vi "Load-Save Color Palette List.vi"(6 "Load (F)/Save":bool, 8 "error in (no error)":errorcluster, 9 "[Color Palette Name] in":string[](array[string]), 10 "Color Palette Target":string="Color Lists", 11 "ini File Refnum in":T1) -> (0 "error out":errorcluster, 1 "[Color Palette Name] out":string[](array[string]), 3 "ini File Refnum out":T1)   [LabVIEW 2021, in "Palette.lvlib"]
uses:
  <vilib>/Utility/config.llb/Config Data RefNum.ctl
  Palette.lvlib
  Variant/Variant to Data/Variant to [String].vi
  <userlib>/_OpenG.lib/variantconfig/variantconfig.llb/openg_variant_configuration_file.lvlib
  Variant/Variant to Data/Variant to Data.lvlib
  <vilib>/Utility/config.llb/NI_LVConfig.lvlib
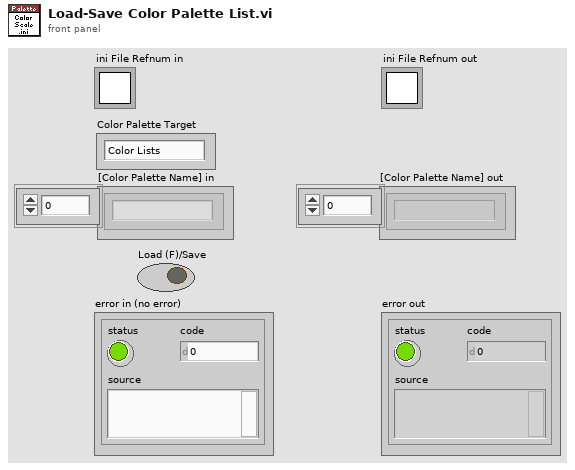
[diagram p1: front panel]
types:
  T1 = typedef "NI_LVConfig.lvlib/Config Data RefNum.ctl" = refnum<k1>
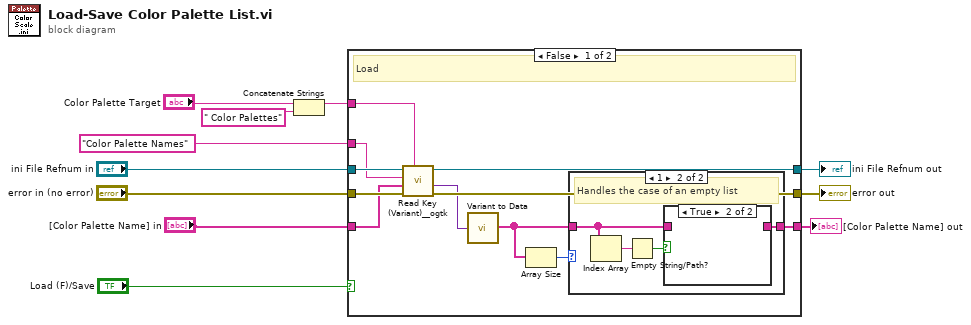
[diagram p0: block diagram]
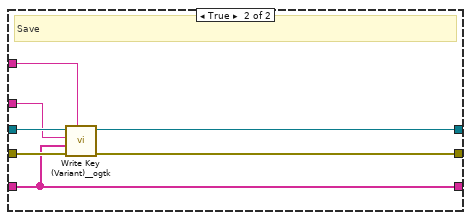
[diagram p4: hidden frame]
diagram:
  n1 = Concatenate Strings("Color Palette Target", " Color Palettes" ("string")) -> (w2:string)
  n2 = case shown="False" "Load (F)/Save" {
    tunnel: "ini File Refnum in" -> [w22 w35]
    tunnel: [w19 w34] -> w8
    tunnel: [w18 w33] -> w6
    tunnel: "error in (no error)" -> [w21 w30]
    tunnel: w2 -> [w17 w32]
    tunnel: "Color Palette Names" ("key (optional)") -> [w20 w31]
    tunnel: "[Color Palette Name] in" -> [w16 w29]
    tunnel: [w12 w29] -> w3
    frame False {
      # "Load"
      n3 = call <userlib>:"Read Key (Variant)__ogtk.vi"("section"=w17, "error in (no error)"=w21, "type"=w16, "key (optional)"=w20, "refnum"=w22) -> ("error out"=w18:errorcluster, "key-value"=w15:variant, "refnum out"=w19:T1)  [unwired: 3 in, 1 out]
      n4 = call-poly "Variant to Data.vi"("Variant"=w15) -> ("String Array"=w13:string[])  [unwired: 8 in]
      n5 = Array Size(array=w13) -> (size(s)=w14:i32)
      n6 = case shown="1" w14 {
        tunnel: w13 -> [w23 w25]
        tunnel: [w23 w24] -> w12
        frame 0, Default {
        }
        frame 1 {
          # "Handles the case of an empty list"
          n7 = Index Array(array=w25) -> (element=w27:string)  [unwired: 1 in]
          n8 = Empty String/Path?(string/path=w27) -> (empty?=w26:bool)
          n9 = case shown="True" w26 {
            tunnel: w25 -> [w28 _]
            tunnel: [w28 _] -> w24
            frame False {
            }
            frame True {
            }
          }
        }
      }
    }
    frame True {
      # "Save"
      n10 = call <userlib>:"Write Key (Variant)__ogtk.vi"("section"=w32, "error in (no error)"=w30, "key-value"=w29, "key (optional)"=w31, "refnum"=w35) -> ("error out"=w33:errorcluster, "refnum out"=w34:T1)  [unwired: 5 in]
    }
  }
  "ini File Refnum out" <- w8
  "error out" <- w6
  "[Color Palette Name] out" <- w3
